vi "Read Line.vi"(8 "error in":errorcluster, 9 "Previous":string, 11 "VISA resource name":refnum<visa-resource-name>) -> (0 "error out":errorcluster, 1 "Remaining":string, 2 "Message":string, 3 "VISA resource name out":refnum<visa-resource-name>)   [LabVIEW 2019, in "Andeen-Hagerling 2700(400 firmware).lvlib"]
doc: "Read a line from the selected VISA resource. Line terminates at the line feed character."
uses:
  Andeen-Hagerling 2700(400 firmware).lvlib
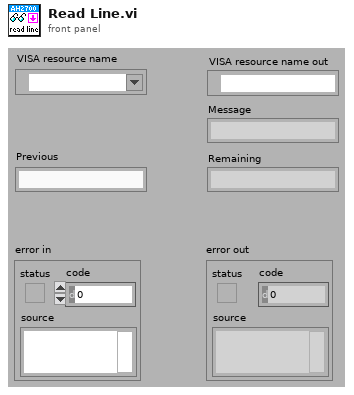
[diagram p1: front panel]
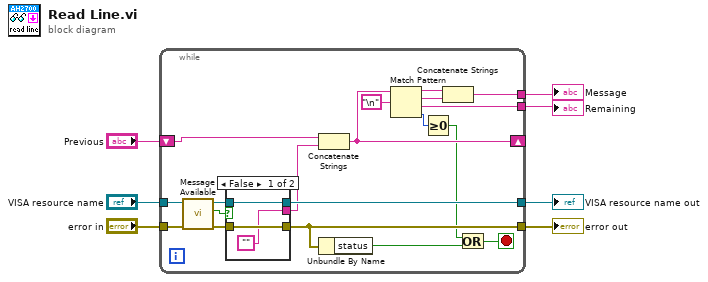
[diagram p0: block diagram]
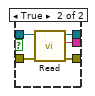
[diagram p2: hidden frame]
diagram:
  n1 = while {
    tunnel: "error in" -> [w26]
    tunnel: "VISA resource name" -> [w25]
    tunnel: [w20] -> w5
    tunnel: [w21] -> w4
    shift-right: [w17] -> _
    shift-left: "Previous" -> [w18]
    tunnel: [w9] -> w2
    tunnel: [w8] -> w3
    stop <- w12 stop-if-true
    n2 = call "Message Available.vi"("error in"=w26, "VISA resource name"=w25) -> ("error out"=w22:errorcluster, "message available"=w24:bool, "VISA resource name out"=w23:refnum<visa-resource-name>)  [unwired: 7 in]
    n3 = case shown="False" w24 {
      tunnel: w23 -> [w29 w34]
      tunnel: w22 -> [w28 w33]
      tunnel: ["" w32] -> w19
      tunnel: [w29 w31] -> w21
      tunnel: [w28 w30] -> w20
      frame False {
      }
      frame True {
        n4 = call "Read.vi"("error in"=w33, "VISA resource name"=w34) -> ("error out"=w30:errorcluster, "Message"=w32:string, "VISA resource name out"=w31:refnum<visa-resource-name>)  [unwired: 7 in]
      }
    }
    n5 = Concatenate Strings(w18, w19) -> (w17:string)
    n6 = Unbundle By Name(w20) -> ("status"=w13:bool)
    n7 = Match Pattern(string=w17, regular expression="\n") -> (before substring=w11:string, match substring=w10:string, after substring=w9:string, offset past match=w15:i32)  [unwired: 1 in]
    n8 = Greater Or Equal To 0?(x=w15) -> (x >= 0?=w14:bool)
    n9 = Concatenate Strings(w11, w10) -> (w8:string)
    n10 = Or(x=w14, y=w13) -> (x .or. y?=w12:bool)
  }
  "VISA resource name out" <- w4
  "error out" <- w5
  "Message" <- w3
  "Remaining" <- w2
